vi "Rectangle To ROI.vi"(8 "error in (no error)":errorcluster, 10 "Global Rectangle in":i32[](array[numeric]), 11 "Camera Prime95B Controller in":refnum<class "CameraController.lvclass">) -> (0 "error out":errorcluster, 2 "Setting.ROI":T1, 3 "Camera Prime95B Controller out":refnum<class "CameraController.lvclass">)   [LabVIEW 2020, in "CameraController.lvlib" / "CameraController.lvclass"]
uses:
  CameraController.lvclass
  CameraController.lvclass/CameraController.ctl
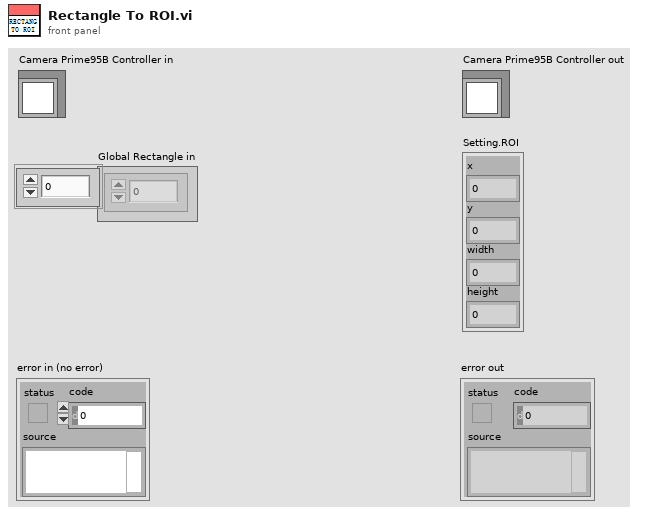
[diagram p1: front panel]
types:
  T1 = cluster{"x":dbl, "y":dbl, "width":dbl, "height":dbl}
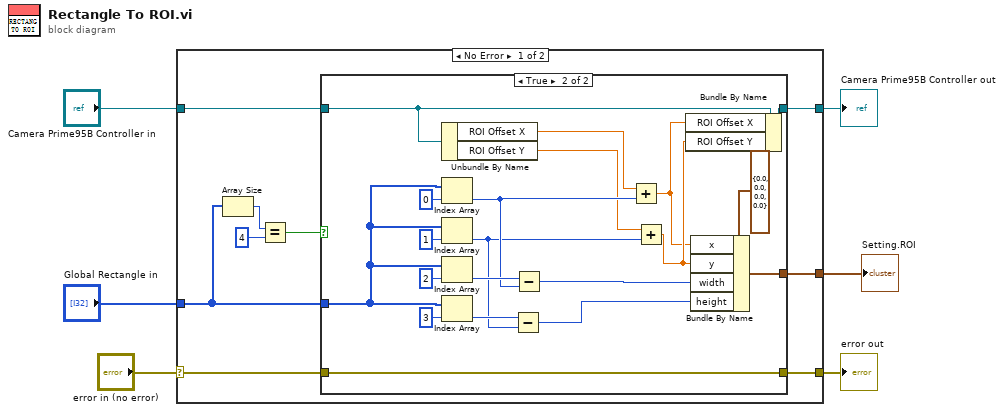
[diagram p0: block diagram]
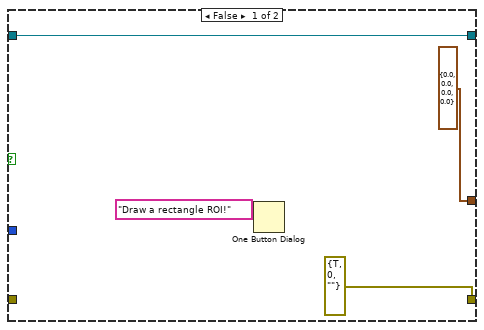
[diagram p2: hidden frame]
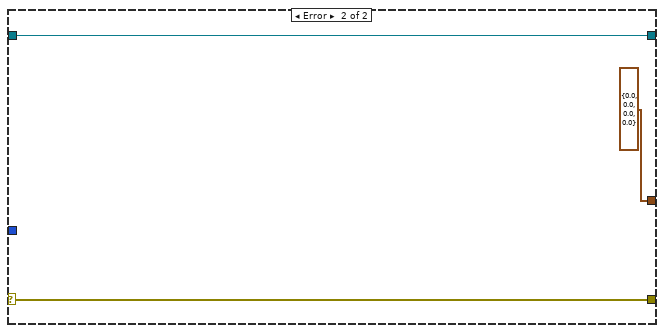
[diagram p3: hidden frame]
diagram:
  n1 = case shown="No Error" "error in (no error)" {
    selector: "error in (no error)" -> [w11 w42]
    tunnel: [w10 w42] -> w5
    tunnel: [w7 w41] -> w3
    tunnel: "Camera Prime95B Controller in" -> [w8 w41]
    tunnel: "Global Rectangle in" -> [w13 _]
    tunnel: [w9 T1 {"x"=0.0, "y"=0.0, "width"=0.0, "height"=0.0} ("Setting.ROI")] -> w1
    frame No Error {
      n2 = Array Size(array=w13) -> (size(s)=w15:i32)
      n3 = Equal?(x=w15, y=4) -> (x = y?=w12:bool)
      n4 = case shown="True" w12 {
        tunnel: w13 -> [_ w33]
        tunnel: w11 -> [_ w32]
        tunnel: [errorcluster {"status"=TRUE, "code"=0, "source"=""} ("error IO") w32] -> w10
        tunnel: [T1 {"x"=0.0, "y"=0.0, "width"=0.0, "height"=0.0} ("Setting.ROI") w30] -> w9
        tunnel: w8 -> [w17 w29]
        tunnel: [w17 w22] -> w7
        frame False {
          n5 = One Button Dialog(message="Draw a rectangle ROI!") -> ()  [unwired: 1 in, 1 out]
        }
        frame True {
          n6 = Unbundle By Name(w29) -> ("ROI Offset X"=w28:dbl, "ROI Offset Y"=w26:dbl)
          n7 = Index Array(array=w33, index=0) -> (element=w27:i32)
          n8 = Index Array(array=w33, index=1) -> (element=w25:i32)
          n9 = Index Array(array=w33, index=2) -> (element=w35:i32)
          n10 = Index Array(array=w33, index=3) -> (element=w34:i32)
          n11 = Subtract(x=w34, y=w25) -> (x-y=w23:i32)
          n12 = Subtract(x=w35, y=w27) -> (x-y=w24:i32)
          n13 = Add(x=w28, y=w27) -> (x+y=w20:dbl)
          n14 = Add(x=w26, y=w25) -> (x+y=w21:dbl)
          n15 = Bundle By Name(cluster=w29, "ROI Offset X"=w20, "ROI Offset Y"=w21) -> (w22:refnum<class "CameraController.lvclass">)
          n16 = Bundle By Name(cluster=T1 {"x"=0.0, "y"=0.0, "width"=0.0, "height"=0.0} ("Setting.ROI"), "x"=w20, "y"=w21, "width"=w24, "height"=w23) -> (w30:T1)
        }
      }
    }
    frame Error {
    }
  }
  "error out" <- w5
  "Camera Prime95B Controller out" <- w3
  "Setting.ROI" <- w1
